vi "CLD 12 CSV file commands utility.vi"(8 "Error In":errorcluster) -> (0 "Error Out":errorcluster, 3 "Command Array Out":T1[](array[typedef]))   [LabVIEW 2019]
doc: "CLD 12: File access utility. This VI converts the text command to the enum equivalent."
uses:
  Controls/CLD 12 Data Cluster.ctl
  Controls/CLD 12 Sequencer Enum.ctl
  <vilib>/Utility/file.llb/Read Delimited Spreadsheet (string).vi
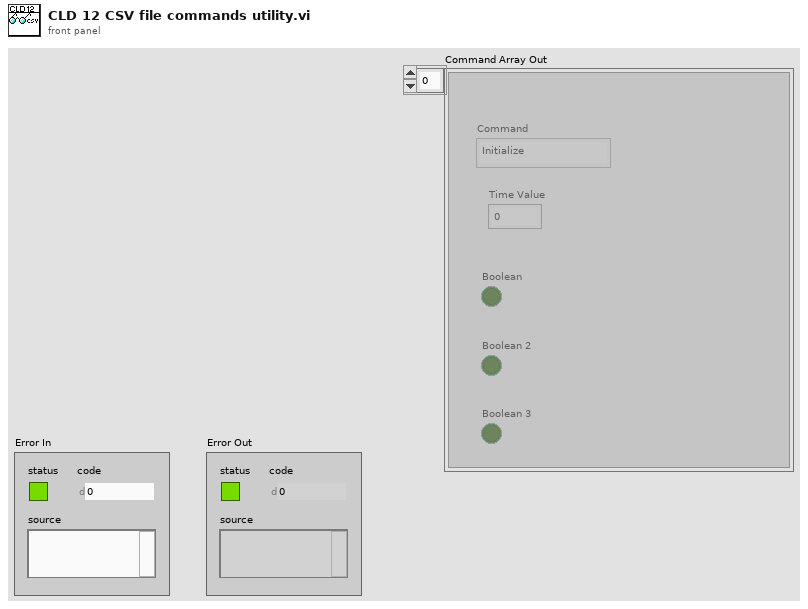
[diagram p1: front panel]
types:
  T1 = typedef "CLD 12 Data Cluster.ctl" = cluster{"Command":T2, "Time Value":dbl, "Boolean":bool, "Boolean 2":bool, "Boolean 3":bool}
  T2 = typedef "CLD 12 Sequencer Enum.ctl" = enum16{"Initialize", "SetTime", "RunState1", "Runstate2", "Idle", "Start"}
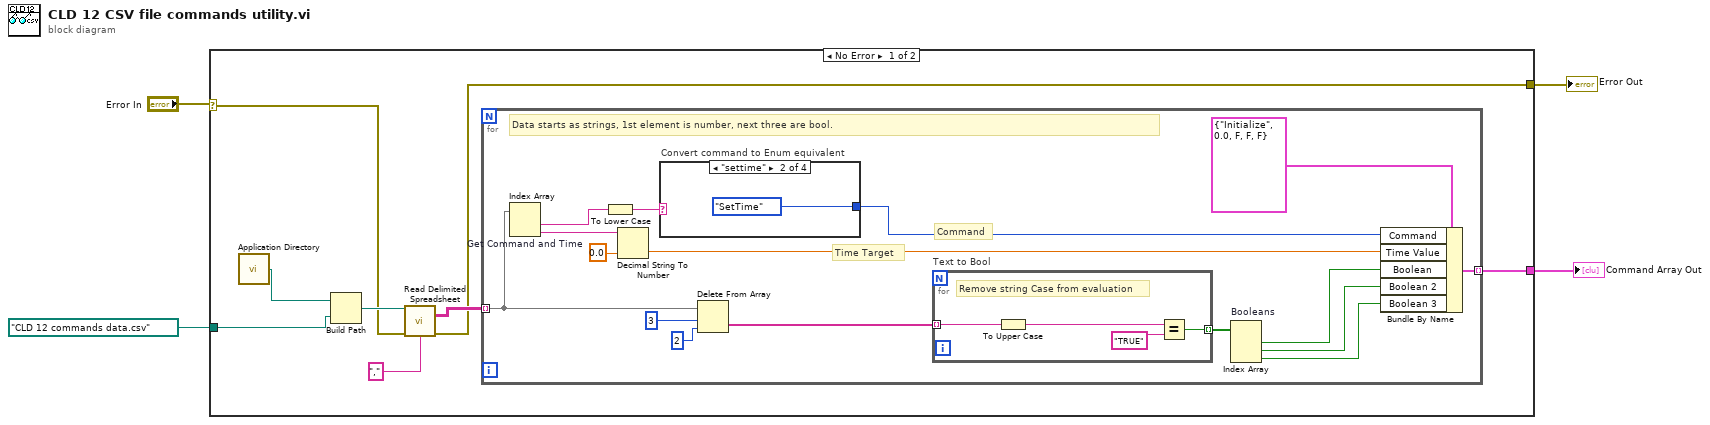
[diagram p0: block diagram]
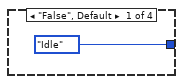
[diagram p2: hidden frame]
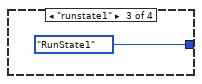
[diagram p3: hidden frame]
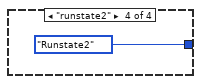
[diagram p4: hidden frame]
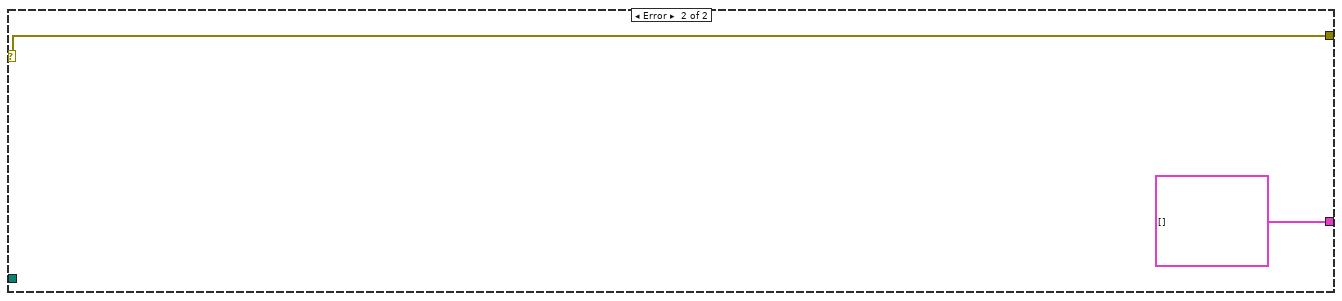
[diagram p5: hidden frame]
diagram:
  n1 = case shown="No Error" "Error In" {
    selector: "Error In" -> [w7 w38]
    tunnel: [w11 T1[] []] -> w1
    tunnel: path "CLD 12 commands data.csv" -> [w10 _]
    tunnel: [w6 w38] -> w2
    frame No Error {
      n2 = call <vilib>:"Application Directory.vi"() -> ("Application Directory"=w5:path)
      n3 = Build Path(base path=w5, name or relative path=w10) -> (appended path=w9:path)
      n4 = call-poly <vilib>:"Read Delimited Spreadsheet.vi"("file path (dialog if empty)"=w9, "error in (no error)"=w7, "delimiter (\\t)"="," ("delimiter (\\t)")) -> ("all rows"=w8:string[][], "error out"=w6:errorcluster)  [unwired: 7 in, 4 out]
      n5 = for {
        tunnel: w8 -> [w28] mode=indexing
        tunnel: [w20] -> w11 mode=indexing
        # "Time Target"
        # "Command"
        # "Data starts as strings, 1st element is number, next three are bool."
        n6 = Index Array "Get Command and Time"(array=w28) -> (element #1=w16:string, element #2=w19:string)  [unwired: 2 in]
        n7 = To Lower Case(string=w16) -> (all lower case string=w14:string)
        n8 = Decimal String To Number(string=w19, default (0L)=0.0) -> (number=w18:dbl)  [unwired: 1 in, 1 out]
        n9 = case "Convert command to Enum equivalent" shown="\"settime\"" w14 {
          tunnel: [CLD_12_Sequencer_Enum."Idle" ("Command") CLD_12_Sequencer_Enum."SetTime" ("Command") CLD_12_Sequencer_Enum."RunState1" ("Command") CLD_12_Sequencer_Enum."Runstate2" ("Command")] -> w15
          frame "False", Default {
          }
          frame "settime" {
          }
          frame "runstate1" {
          }
          frame "runstate2" {
          }
        }
        n10 = Delete From Array(array=w28, length=3, index=2) -> (deleted portion=w13:string[])  [unwired: 1 out]
        n11 = for "Text to Bool" {
          tunnel: w13 -> [w32] mode=indexing
          tunnel: [w29] -> w25 mode=indexing
          # "Remove string Case from evaluation"
          n12 = To Upper Case(1:w32) -> (0:w31:string)
          n13 = Equal?(x=w31, y="TRUE") -> (x = y?=w29:bool)
        }
        n14 = Index Array "Booleans"(array=w25) -> (element #1=w23:bool, element #2=w22:bool, element #3=w21:bool)  [unwired: 3 in]
        n15 = Bundle By Name(cluster=T1 {"Command"=enum."Initialize", "Time Value"=0.0, "Boolean"=FALSE, "Boolean 2"=FALSE, "Boolean 3"=FALSE} ("CLD 12 Data Cluster"), "Command"=w15, "Time Value"=w18, "Boolean"=w23, "Boolean 2"=w22, "Boolean 3"=w21) -> (w20:T1)
      }
    }
    frame Error {
    }
  }
  "Error Out" <- w2
  "Command Array Out" <- w1
